vi "SL_Control.vi"(0 "Elapsed Time (s)":dbl, 5 "Previous Time In":dbl caption="Previous Time In (s)", 7 "Timer In":dbl caption="Timer In (s)", 9 "Period":dbl caption="Period (s)", 11 "Amplitude (sscm)":dbl, 12 "Debug Mode":bool) -> (4 "Previous Time Out":dbl caption="Previous Time Out (s)", 6 "Timer Out":dbl caption="Timer Out (s)", 8 "Flow":dbl caption="Flow (sscm)")   [LabVIEW 2011]
doc: "This VI controls the flow of Gallium to make it oscillate over a square wave. See the API Programming Guide for more details."
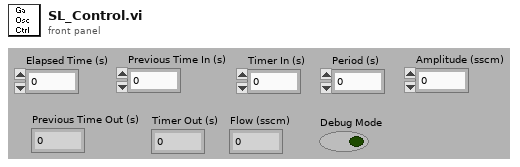
[diagram p1: front panel]
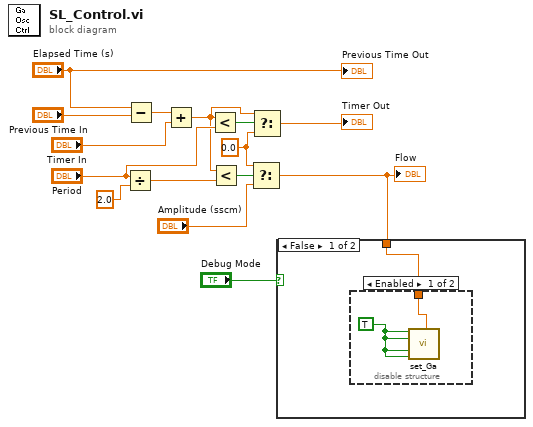
[diagram p0: block diagram]
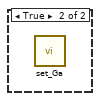
[diagram p3: hidden frame]
diagram:
  w4 = 0.0 ("t")
  n1 = Divide(x="Period", y=2.0) -> (x/y=w12:dbl)
  n2 = Subtract(x="Elapsed Time (s)", y="Previous Time In") -> (x-y=w14:dbl)
  n3 = Add(x=w14, y="Timer In") -> (x+y=w5:dbl)
  n4 = Less?(x=w5, y="Period") -> (x < y?=w6:bool)
  n5 = Less?(x=w5, y=w12) -> (x < y?=w11:bool)
  n6 = Select(t=w4, s=w11, f="Amplitude (sscm)") -> (s? t:f=w1:dbl)
  "Flow" <- w1
  n7 = Select(t=w5, s=w6, f=w4) -> (s? t:f=→"Timer Out":dbl)
  n8 = case shown="False" "Debug Mode" {
    tunnel: w1 -> [w16 _]
    frame False {
      n9 = disable-structure shown="Enabled" {
        disable-tunnel: w16 -> [w18 _]
        frame Enabled {
          w17 = TRUE ("Ga Active")
          n10 = call "set_Ga.vi"("Ga Active"=w17, "Ga Flow 1"=w18, "Ga Bubbler"=w17, "Ga Run"=w17, "Ga Remote"=w17) -> ()  [unwired: 3 in, 8 out]
        }
        frame Disabled {
        }
      }
    }
    frame True {
      n11 = call "set_Ga.vi"() -> ()  [unwired: 8 in, 8 out]
    }
  }
  "Previous Time Out" <- "Elapsed Time (s)"
